vi "New sensor.vi"(11 "error in (no error)":errorcluster) -> (3 "error out":errorcluster)   [LabVIEW 2019]
uses:
  <vilib>/myRIO/Instrument Drivers/Onboard IO/DIO/typedefs/DIO Reference.ctl
  <vilib>/myRIO/Common/Instrument Driver Framework/Utilities/typedefs/myRIO Generic Hardware Reference.ctl
  <vilib>/myRIO/Common/Instrument Driver Framework/Utilities/typedefs/Hardware Version Enum.ctl
  <vilib>/myRIO/Common/Instrument Driver Framework/Utilities/typedefs/myRIO v1.0 Reference.ctl
  <vilib>/myRIO/Common/Instrument Driver Framework/Utilities/typedefs/Generic FPGA Reference.ctl
  <vilib>/myRIO/Common/Instrument Driver Framework/myRIO v1.0/DIO/typedefs/DIO Channels List.ctl
  <vilib>/myRIO/Common/Instrument Driver Framework/myRIO v1.0/DIO/typedefs/DIO Channels Enum.ctl
  <vilib>/userdefined/High Color/nirio_resource_hc.ctl
  <vilib>/myRIO/Instrument Drivers/Onboard IO/I2C/typedefs/I2C User Configuration.ctl
  <vilib>/myRIO/Instrument Drivers/Onboard IO/I2C/typedefs/I2C Transfer Rate.ctl
  <vilib>/myRIO/Instrument Drivers/Onboard IO/I2C/typedefs/I2C Reference.ctl
  <vilib>/myRIO/Common/Instrument Driver Framework/myRIO v1.0/I2C/typedefs/I2C Channels Enum.ctl
  <vilib>/myRIO/Instrument Drivers/Onboard IO/I2C/typedefs/I2C Configuration.ctl
  <vilib>/Platform/TimedLoop/XDataNode/timing_clust.ctl
  <vilib>/Platform/TimedLoop/XDataNode/nitl_modes.ctl
  <vilib>/Platform/TimedLoop/XDataNode/wakeup.ctl
  <vilib>/myRIO/Common/Instrument Driver Framework/Utilities/vis/Is FPGA Ref Available.vi
  <vilib>/myRIO/Common/Instrument Driver Framework/myRIO v1.0/DIO/vis/myRIO v1.1 Open DIO.vi
  <vilib>/myRIO/Instrument Drivers/Onboard IO/DIO/vis/Write.vi
  <vilib>/myRIO/Common/Instrument Driver Framework/myRIO v1.0/I2C/vis/myRIO v1.1 Open I2C.vi
  <vilib>/myRIO/Instrument Drivers/Onboard IO/I2C/vis/Configure.vi
  <vilib>/myRIO/Instrument Drivers/Onboard IO/I2C/vis/Write.vi
  <vilib>/myRIO/Instrument Drivers/Onboard IO/I2C/vis/Read.vi
  <vilib>/myRIO/Common/Instrument Driver Framework/Utilities/vis/Validate Channels.vi
  <vilib>/myRIO/Common/Instrument Driver Framework/myRIO v1.0/DIO/vis/myRIO v1.0 Reserve DIO.vi
  <vilib>/myRIO/Common/Instrument Driver Framework/myRIO v1.0/I2C/vis/myRIO v1.0 Reserve I2C.vi
  <vilib>/myRIO/Common/Instrument Driver Framework/myRIO v1.0/Resource Manager/vis/myRIO v1.0 Reserve Channel List.vi
  <vilib>/myRIO/Common/Instrument Driver Framework/myRIO v1.0/DIO/vis/myRIO v1.0 Build MUX Configuration DIO.vi
  <vilib>/myRIO/Common/Instrument Driver Framework/myRIO v1.0/I2C/vis/myRIO v1.0 Build MUX Configuration I2C.vi
  <vilib>/myRIO/Common/Instrument Driver Framework/myRIO v1.0/Resource Manager/vis/myRIO v1.0 Reserve Channel.vi
  <vilib>/myRIO/Common/Instrument Driver Framework/myRIO v1.0/Resource Manager/vis/myRIO v1.0 Unreserve Channel.vi
  <vilib>/myRIO/Common/Instrument Driver Framework/myRIO v1.0/Resource Manager/vis/myRIO v1.0 Create Configuration List.vi
  <vilib>/myRIO/Common/Instrument Driver Framework/myRIO v1.0/Resource Manager/vis/myRIO v1.0 Build Mutex Name.vi
  <vilib>/Utility/VariantDataType/GetNumericInfo.vi
  <vilib>/Utility/error.llb/Error Cluster From Error Code.vi
  <vilib>/myRIO/Common/Instrument Driver Framework/myRIO v1.0/myRIO v1.1 Open.vi
  <vilib>/myRIO/Common/Instrument Driver Framework/Utilities/vis/IO Manager.vi
  <vilib>/myRIO/Common/Instrument Driver Framework/Utilities/vis/Configuration Manager.vi
  <vilib>/myRIO/Common/Instrument Driver Framework/myRIO v1.0/Resource Manager/vis/myRIO v1.0 Configure IO.vi
  <vilib>/myRIO/Common/Instrument Driver Framework/myRIO v1.0/myRIO v1.0 Close.vi
  <vilib>/myRIO/Common/Instrument Driver Framework/myRIO v1.0/DIO/vis/myRIO v1.0 Write DIO.vi
  <vilib>/myRIO/Common/Instrument Driver Framework/myRIO v1.0/I2C/vis/myRIO v1.0 Configure I2C.vi
  <vilib>/myRIO/Common/Instrument Driver Framework/myRIO v1.0/I2C/vis/myRIO v1.0 Write I2C.vi
  Global.vi
  <vilib>/myRIO/Common/Instrument Driver Framework/myRIO v1.0/I2C/vis/myRIO v1.0 Read I2C.vi
  <vilib>/myRIO/Express VI/Onboard IO/DO/DO Express VI.xnode
  <vilib>/myRIO/Instrument Drivers/Onboard IO/DIO/vis/myRIO DIO Open.xnode
  <vilib>/myRIO/Express VI/Onboard IO/I2C/I2C Express VI.xnode
  <vilib>/myRIO/Instrument Drivers/Onboard IO/I2C/vis/myRIO I2C Open.xnode
  <vilib>/platform/TimedLoop/XDataNode/XDataNode.xnode
  <vilib>/Platform/TimedLoop/XDataNode/XDNodeRunTimeDep.lvlib
  <vilib>/Analysis/NI_AAL_SigProc.lvlib
  <vilib>/ptbypt/NI_PtbyPt.lvlib
  <vilib>/myRIO/Instrument Drivers/Onboard IO/I2C/I2C.lvlib
  <vilib>/myRIO/Instrument Drivers/Onboard IO/DIO/DIO.lvlib
panel:
  in  "Tab Control 2":enum32{"Graph", "Filter controls"}(tab)
  out "Sensors data":T1(graph)
  in  "Sensor Tare":bool
  in  "Tare sensor 1":dbl
  in  "Tare reset val":dbl=-44.0
  out "element old":dbl
  in  "Width":i32(slide)=10 scale=0.0..500.0
  in  "Threshold":dbl(slide)=4.897959183673464 scale=-60.0..60.0
  out "Locations":dbl[](array[numeric])
  out "element":dbl
  out "size(s)":i32
  in  "Ts":dbl=0.01
  in  "Tf":dbl=0.001 format="%#_13g"
  in  "Tf 2":dbl=0.8
  in  "Ts 2":dbl=0.01
  in  "sample length":i32=50
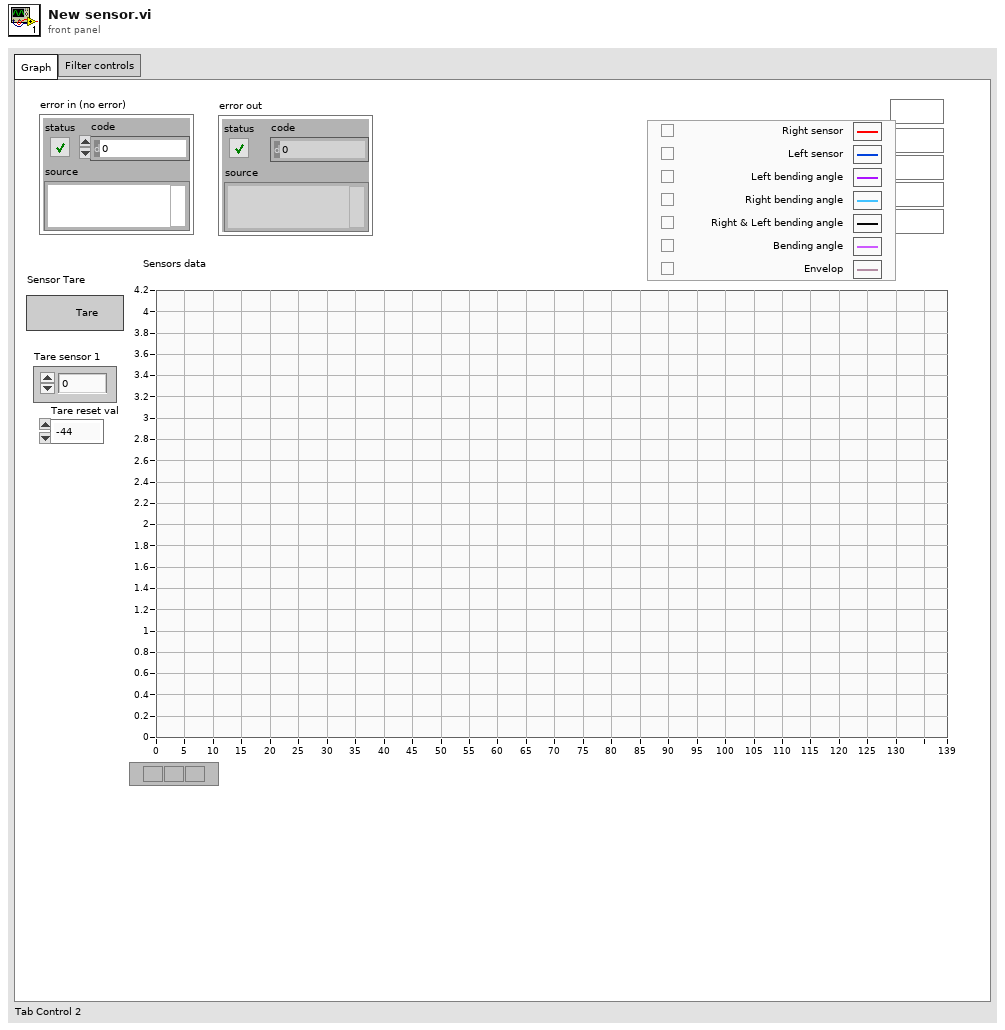
[diagram p1: front panel]
types:
  T1 = cluster{dbl, "yf1":dbl, "yf1":dbl, "mean":dbl, dbl}
  T2 = cluster{dbl, "yf1":dbl, "yf1":dbl, "mean":dbl, dbl}[]
  T3 = typedef "DIO.lvlib/DIO Reference.ctl" = cluster{"myRIO Reference":T4, "DIO Channels List":T8}
  T4 = typedef "myRIO Generic Hardware Reference.ctl" = cluster{"myRIO Model":T5, "myRIO Hardware Reference":T6}
  T5 = typedef "Hardware Version Enum.ctl" = enum16{"Unknown", "myRIO-1900", "myRIO-1950", "roboRIO", "NI ELVIS RIO CM", "ELVIS III"}
  T6 = typedef "myRIO v1.0 Reference.ctl" = cluster{"Generic FPGA Reference":T7, "Allow multiple opens":bool}
  T7 = typedef "Generic FPGA Reference.ctl" = refnum<k20>
  T8 = typedef "DIO Channels List.ctl" = T9[]
  T9 = typedef "DIO Channels Enum.ctl" = enum16{"Not Connected", "C/DIO0", "C/DIO1", "C/DIO2", "C/DIO3", "C/DIO4", "C/DIO5", "C/DIO6", "C/DIO7", "A/DIO0", "A/DIO1", "A/DIO2", "A/DIO3", "A/DIO4", "A/DIO5", "A/DIO6", "A/DIO7", "A/DIO8", "A/DIO9", "A/DIO10", "A/DIO11", "A/DIO12", "A/DIO13", "A/DIO14", "A/DIO15", "A/DIO16", "A/DIO17", "A/DIO18", "A/DIO19", "B/DIO0", "B/DIO1", "B/DIO2", "B/DIO3", "B/DIO4", "B/DIO5", "B/DIO6", "B/DIO7", "B/DIO8", "B/DIO9", "B/DIO10", "B/DIO11", "B/DIO12", "B/DIO13", "B/DIO14", "B/DIO15", "B/DIO16", "B/DIO17", "B/DIO18", "B/DIO19", "LED0", "LED1", "LED2", "LED3", "Button0", "DIO/DIO0", "DIO/DIO1", "DIO/DIO2", "DIO/DIO3", "DIO/DIO4", "DIO/DIO5", "DIO/DIO6", "DIO/DIO7", "DIO/DIO8", "DIO/DIO9", "SPI/CS0", "SPI/CS1", "SPI/CS2", "SPI/CS3", "LED RADIO (Green)", "LED RADIO (Red)", "LED COMM (Green)", "LED COMM (Red)", "LED MODE (Green)", "LED MODE (Red)"}
  T10 = typedef "nirio_resource_hc.ctl" = tag
  T11 = typedef "I2C.lvlib/I2C Reference.ctl" = cluster{"myRIO Reference":T4, "I2C Channels Enum":T12, "I2C Configuration":T13}
  T12 = typedef "I2C Channels Enum.ctl" = enum16{"Not Connected", "A/I2C", "B/I2C", "I2C/I2C"}
  T13 = typedef "I2C.lvlib/I2C Configuration.ctl" = cluster{"I2C Transfer Rate":T14}
  T14 = typedef "I2C.lvlib/I2C Transfer Rate.ctl" = enum16{"Standard mode (100 kbps)", "Fast mode (400 kbps)"}
  T15 = typedef "I2C.lvlib/I2C User Configuration.ctl" = cluster{"I2C Transfer Rate":T14}
  T16 = typedef "XDNodeRunTimeDep.lvlib/timing_clust.ctl" = cluster{"Expected End [f-1]":u64, "Actual End [f-1]":u64, "Finished Late? [f-1]":bool, "Expected End [i-1]":u64, "Actual End [i-1]":u64, "Finished Late? [i-1]":bool, "Expected Start [i]":u64, "Actual Start [i]":u64, "Expected Start [f]":u64, "Actual Start [f]":u64, "Source Name":string, "Structure Name":string, "Period":i64, "Deadline":i64, "Offset":i64, "Start":i64, "Priority":i32, "Timeout":i32, "Mode":T17, "Wakeup Reason":T18, "Error":errorcluster, "Source Type":string, "Secondary Source Type":string, "Global End Time":u64, "Global Start Time":u64, "Frame Duration":u64, "Iteration Duration":u64, "Assigned CPU":i32, "I/O Scan Engine Mode":u32}
  T17 = typedef "XDNodeRunTimeDep.lvlib/nitl_modes.ctl" = enum32{"No Change", "Process missed periods, maintain original phase", "Discard missed periods, maintain original phase", "Process missed periods, ignore original phase", "Discard missed periods, ignore original phase"}
  T18 = typedef "XDNodeRunTimeDep.lvlib/wakeup.ctl" = enum32{"Normal", "Aborted", "Asynchronous wakeup", "Timing source error", "Timed loop error", "Timeout"}
  T19 = cluster{dbl, "yf1":dbl, "yf1":dbl, "mean":dbl, "yf":dbl}
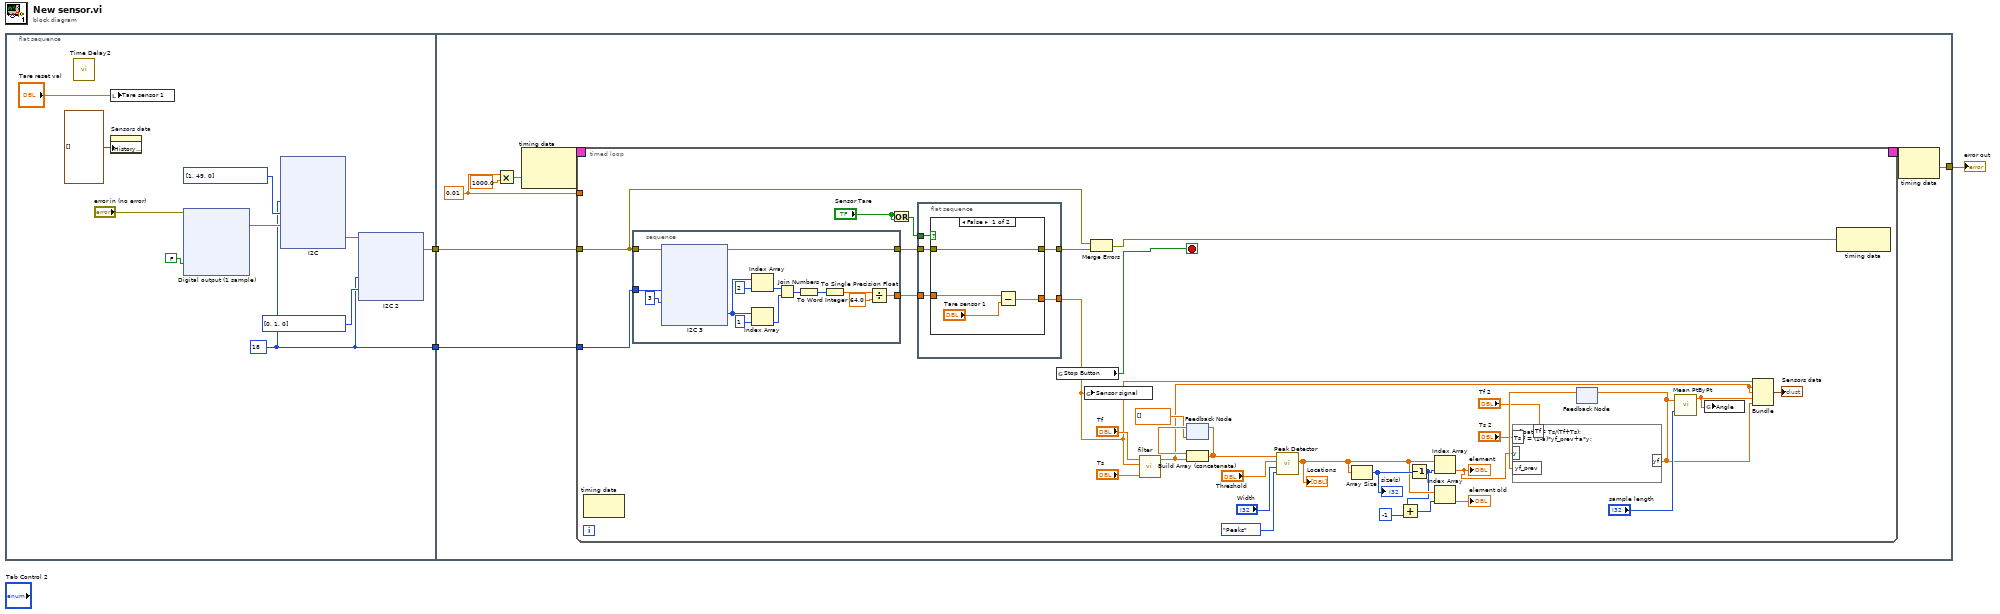
[diagram p0: block diagram]
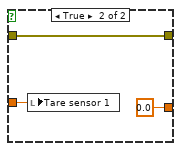
[diagram p2: hidden frame]
diagram:
  n1 = flat-sequence {
    tunnel: [w8] -> w3
    tunnel: [w6] -> w2
    tunnel: w3 -> [w126]
    tunnel: w2 -> [w127]
    tunnel: [w125] -> w1
    frame #0 {
      w8 = u8 18 ("Slave Address (7-bit)")
      n2 = call "Time Delay2"() -> ()  [unwired: 11 in, 1 out]
      n3 = local write "Tare sensor 1"("Tare reset val") -> ()
      n4 = property on="Sensors data" class="WFChart (strict)"("History Data"=T2 []) -> ()  [unwired: 2 in, 2 out]
      n5 = xnode "Digital output (1 sample)"("A/DIO10 (Pin 31)"=FALSE, "error in (no error)"="error in (no error)") -> ("error out"=w9:errorcluster)
      n6 = xnode "I2C"("Slave Address (7-bit)"=w8, "Bytes to Write"=u8[] [1, 49, 0], "error in (no error)"=w9) -> ("error out"=w12:errorcluster)
      n7 = xnode "I2C 2"("Slave Address (7-bit)"=w8, "Bytes to Write"=u8[] [0, 1, 0], "error in (no error)"=w12) -> ("error out"=w6:errorcluster)
    }
    frame #1 {
      w128 = 0.01
      n8 = Multiply(x=w128, y=1000.0) -> (x*y=w129:dbl)
      n9 = node-c288(w129) -> (w132:T16)  [unwired: 1 in]
      n10 = timed-loop {
        tunnel: w127 -> [w141]
        timing: w132 -> [_]
        timing-out: [_] -> w131
        tunnel: w128 -> [_]
        tunnel: w126 -> [w151]
        stop <- w140 stop-if-true
        n11 = node-c288() -> ()  [unwired: 1 in, 1 out]
        n12 = stacked-sequence {
          tunnel: [w184] -> w165
          tunnel: w141 -> [w185]
          tunnel: w151 -> [w183]
          tunnel: [w182] -> w145
          frame #0 {
            n13 = xnode "I2C 3"("Slave Address (7-bit)"=w183, "Byte Count"=u32 3, "error in (no error)"=w185) -> ("Bytes Read"=w186:u8[], "error out"=w182:errorcluster)
            n14 = Index Array(array=w186, index=2) -> (element=w187:u8)
            n15 = Index Array(array=w186, index=1) -> (element=w188:u8)
            n16 = Join Numbers(hi=w187, lo=w188) -> ((hi.lo)=w189:u16)
            n17 = To Word Integer(number=w189) -> (16bit integer=w190:i16)
            n18 = To Single Precision Float(number=w190) -> (single precision float=w191:sgl)
            n19 = Divide(x=w191, y=sgl 64.0) -> (x/y=w184:sgl)
          }
        }
        n20 = Or(x="Sensor Tare", y="Sensor Tare") -> (x .or. y?=w143:bool)
        n21 = flat-sequence {
          tunnel: [w174] -> w147
          tunnel: w165 -> [w173]
          tunnel: w145 -> [w172]
          tunnel: [w171] -> w144
          tunnel: w143 -> [w170]
          frame #0 {
            n22 = case shown="False" w170 {
              tunnel: [w178 0.0] -> w174
              tunnel: w173 -> [w177 w180]
              tunnel: w172 -> [w175 w179]
              tunnel: [w175 w179] -> w171
              frame False {
                n23 = Subtract(x=w177, y="Tare sensor 1") -> (x-y=w178:dbl)
              }
              frame True {
                n24 = local write "Tare sensor 1"(w180) -> ()
              }
            }
          }
        }
        n25 = global read "Global.vi" "Stop Button"() -> (w140:bool)
        n26 = global write "Global.vi" "Sensor signal"(w147) -> ()
        n27 = Merge Errors(w141, w144) -> (w148:errorcluster)
        n28 = call "filter.vi"("Ts"="Ts", "y1"=w147, "Tf"="Tf") -> ("yf1"=w139:dbl)  [unwired: 7 in, 1 out]
        n29 = feedback #1(dbl[] []) -> (w162:dbl[])
        n30 = Build Array (concatenate)(w162, w139) -> (w157:dbl[])
        n31 = feedback-in #1(w157) -> ()
        n32 = call <vilib>:"Peak Detector.vi"("peaks/valleys"=enum32{"Peaks", "Valleys"}."Peaks", "width"="Width", "threshold"="Threshold", "X"=w157) -> ("Amplitudes"=w138:dbl[])  [unwired: 3 in, 4 out]
        "Locations" <- w138
        n33 = Array Size(array=w138) -> (size(s)=w156:i32)
        "size(s)" <- w156
        n34 = Decrement(x=w156) -> (x-1=w136:i32)
        n35 = Add(x=w136, y=-1) -> (x+y=w137:i32)
        n36 = Index Array(array=w138, index=w136) -> (element=w134:dbl)
        "element" <- w134
        n37 = Index Array(array=w138, index=w137) -> (element=→"element old":dbl)
        n38 = feedback #2() -> (w155:dbl)  [unwired: 1 in]
        n39 = formula code="float a = Ts/(Tf+Ts);\nyf = (1-a)*yf_prev+a*y;"("Tf"="Tf 2", "Ts"="Ts 2", "y"=w134, "yf_prev"=w155) -> ("yf"=w146:dbl)
        n40 = feedback-in #2(w146) -> ()
        n41 = call <vilib>:"Mean PtByPt.vi"("x"=w146, "sample length"="sample length") -> ("mean"=w150:dbl)  [unwired: 2 in, 1 out]
        n42 = global write "Global.vi" "Angle"(w150) -> ()
        n43 = Bundle(w147, "yf1"=w139, "yf1"=w139, "mean"=w150, "yf"=w146) -> (→"Sensors data":T19)  [unwired: 1 in]
        n44 = node-c288(w148) -> ()  [unwired: 1 out]
      }
      n45 = node-c288(w131) -> (w125:errorcluster)
    }
  }
  "error out" <- w1
